vi "Plane Fit.vi"(8 "Sensitivity":dbl=3.5, 9 "Z":dbl, 10 "Nano Z":dbl, 11 "X":dbl) -> (2 "Output":dbl, 3 "Clicks":dbl)   [LabVIEW 2017]
uses:
  Program Files/National Instruments/LabVIEW 2019/user.lib/HapticSTM/HapticSTM.lvlib
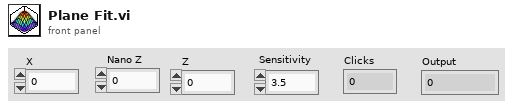
[diagram p1: front panel]
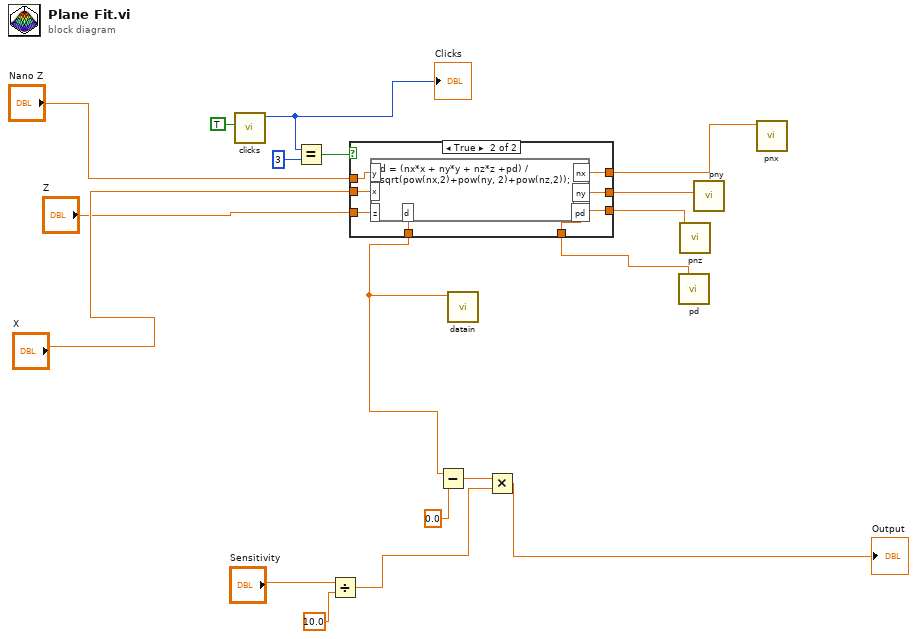
[diagram p0: block diagram]
diagram:
  n1 = call "clicks.vi"("planing"=TRUE) -> ("function return"=w11:i32)  [unwired: 10 in]
  "Clicks" <- w11
  n2 = Equal?(x=w11, y=3) -> (x = y?=w9:bool)
  n3 = Divide(x="Sensitivity", y=10.0) -> (x/y=w17:dbl)
  n4 = call "pd.vi"() -> ("function return"=w12:dbl)  [unwired: 11 in]
  n5 = call "pnz.vi"() -> ("function return"=w13:dbl)  [unwired: 11 in]
  n6 = call "pny.vi"() -> ("function return"=w7:dbl)  [unwired: 11 in]
  n7 = call "pnx.vi"() -> ("function return"=w8:dbl)  [unwired: 11 in]
  n8 = case shown="True" w9 {
    tunnel: "X" -> [_ w27]
    tunnel: [w19 w26] -> w2
    tunnel: w8 -> [_ w25]
    tunnel: w7 -> [_ w24]
    tunnel: w13 -> [_ w23]
    tunnel: w12 -> [_ w22]
    tunnel: "Nano Z" -> [w19 w21]
    tunnel: "Z" -> [_ w20]
    frame False {
    }
    frame True {
      n9 = formula code="d = (nx*x + ny*y + nz*z +pd) / sqrt(pow(nx,2)+pow(ny, 2)+pow(nz,2));"("y"=w21, "z"=w20, "x"=w27, "nx"=w25, "ny"=w24, "nz"=w23, "pd"=w22) -> ("d"=w26:dbl)
    }
  }
  n10 = Subtract(x=w2, y=0.0 ("x")) -> (x-y=w18:dbl)
  n11 = call "datain.vi"("output"=w2) -> ()  [unwired: 11 in]
  n12 = Multiply(x=w18, y=w17) -> (x*y=→"Output":dbl)
